vi "Match Point Clouds.vi"(2 "Reference Offset":cluster{dbl, dbl}, 3 "Centred Reference Points":cluster{dbl[], dbl[]}, 4 "Points to Match Offset":cluster{dbl, dbl}, 5 "Centred Points To Match":cluster{dbl[], dbl[]}) -> (0 "Translation Y":dbl, 1 "Translation X":dbl)   [LabVIEW 2013]
uses:
  <vilib>/Analysis/Matrix/Datatypes/RealMatrix.ctl
  <vilib>/Analysis/Matrix/Numeric/Conversions/Array To Matrix - RA.vi
  <vilib>/Analysis/7linalg.llb/Real SVD Decomposition.vi
  <vilib>/Analysis/Matrix/Numeric/Multiply/Multiply - RM,RM.vi
  <vilib>/Analysis/Matrix/Numeric/Subtract/Subtract - RM,RM.vi
  <vilib>/Analysis/Matrix/Numeric/Add/Add - RM,RM.vi
  <vilib>/Analysis/Matrix/NI_Matrix.lvlib
  <vilib>/Analysis/NI_AALPro.lvlib
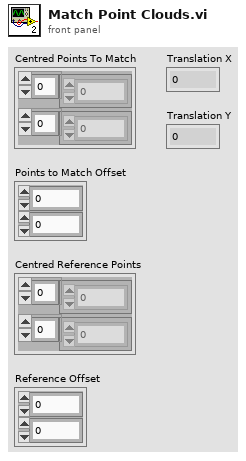
[diagram p1: front panel]
types:
  T1 = typedef "NI_Matrix.lvlib/RealMatrix.ctl" = dbl[][]
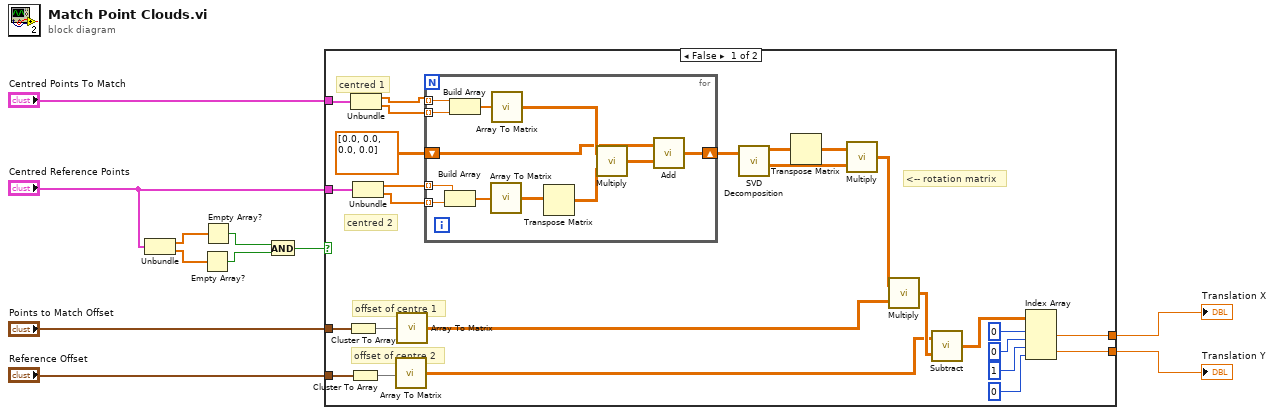
[diagram p0: block diagram]
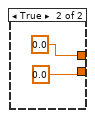
[diagram p2: hidden frame]
diagram:
  n1 = Unbundle("Centred Reference Points") -> (w5:dbl[], w6:dbl[])
  n2 = Empty Array?(array=w6) -> (empty?=w9:bool)
  n3 = Empty Array?(array=w5) -> (empty?=w8:bool)
  n4 = And(x=w8, y=w9) -> (x .and. y?=w10:bool)
  n5 = case shown="False" w10 {
    tunnel: "Centred Points To Match" -> [w21 _]
    tunnel: "Centred Reference Points" -> [w18 _]
    tunnel: [w23 0.0 ("Real Matrix Element")] -> w1
    tunnel: [w22 0.0 ("Real Matrix Element")] -> w2
    tunnel: "Points to Match Offset" -> [w14 _]
    tunnel: "Reference Offset" -> [w12 _]
    frame False {
      # "<-- rotation matrix"
      # "offset of centre 2"
      # "offset of centre 1"
      # "centred 2"
      # "centred 1"
      n6 = Cluster To Array(cluster=w14) -> (array=w15:dbl[])
      n7 = Cluster To Array(cluster=w12) -> (array=w13:dbl[])
      n8 = Unbundle(w21) -> (w20:dbl[], w19:dbl[])
      n9 = Unbundle(w18) -> (w17:dbl[], w16:dbl[])
      n10 = call-poly <vilib>:"Array To Matrix.vi"("Real 1D Array"=w13) -> ("Real Matrix (Column Vector)"=w29:T1)
      n11 = call-poly <vilib>:"Array To Matrix.vi"("Real 1D Array"=w15) -> ("Real Matrix (Column Vector)"=w32:T1)
      n12 = for {
        tunnel: w20 -> [w49] mode=indexing
        tunnel: w19 -> [w48] mode=indexing
        tunnel: w17 -> [w46] mode=indexing
        tunnel: w16 -> [w45] mode=indexing
        shift-right: [w38] -> w36
        shift-left: T1 [[0.0, 0.0], [0.0, 0.0]] ("A * B") -> [w39]
        n13 = Build Array(w46, w45) -> (w44:dbl[])
        n14 = Build Array(w49, w48) -> (w47:dbl[])
        n15 = call-poly <vilib>:"Array To Matrix.vi"("Real 1D Array"=w44) -> ("Real Matrix (Column Vector)"=w43:T1)
        n16 = call-poly <vilib>:"Array To Matrix.vi"("Real 1D Array"=w47) -> ("Real Matrix (Column Vector)"=w41:T1)
        n17 = Transpose Matrix(1:w43) -> (0:w42:T1)
        n18 = call-poly <vilib>:"Multiply.vi"("Real Matrix B"=w42, "Real Matrix A"=w41) -> ("A * B"=w40:T1)
        n19 = call-poly <vilib>:"Add.vi"("Real Matrix B"=w40, "Real Matrix A"=w39) -> ("A + B"=w38:T1)
      }
      n20 = call-poly <vilib>:"SVD Decomposition.vi"("A"=w36) -> ("Matrix V"=w33:T1, "Matrix U"=w35:T1)  [unwired: 6 in, 3 out]
      n21 = Transpose Matrix(1:w35) -> (0:w34:T1)
      n22 = call-poly <vilib>:"Multiply.vi"("Real Matrix B"=w33, "Real Matrix A"=w34) -> ("A * B"=w31:T1)
      n23 = call-poly <vilib>:"Multiply.vi"("Real Matrix B"=w32, "Real Matrix A"=w31) -> ("A * B"=w30:T1)
      n24 = call-poly <vilib>:"Subtract.vi"("Real Matrix B"=w30, "Real Matrix A"=w29) -> ("A - B"=w28:T1)
      n25 = Index Array(array=w28, index (row) #1=0 ("index (row)"), index (col) #1=0 ("index (col)"), index (row) #2=1 ("index (row)"), index (col) #2=0 ("index (col)")) -> (element #1=w23:dbl, element #2=w22:dbl)
    }
    frame True {
    }
  }
  "Translation Y" <- w2
  "Translation X" <- w1
